vi "Set Winding.vi"(11 "Recipes.Winding":T1) -> (3 "concatenated string":string)   [LabVIEW 2014, in "Programing Logic.lvclass"]
uses:
  Programming Logic/Programing Logic.lvclass
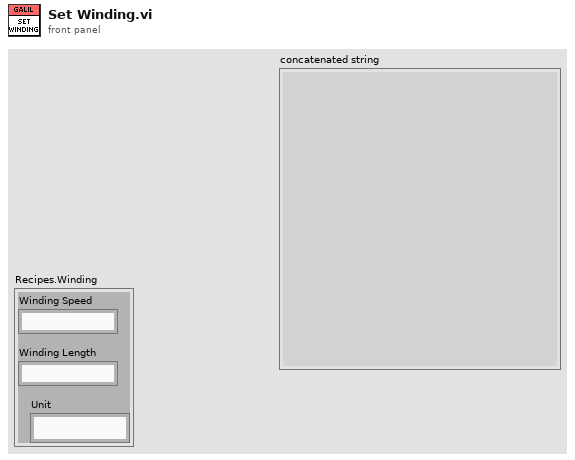
[diagram p1: front panel]
types:
  T1 = cluster{"Winding Speed":string, "Winding Length":string, "Unit":string}
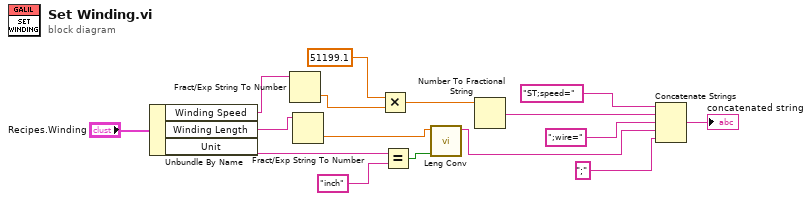
[diagram p0: block diagram]
diagram:
  n1 = Unbundle By Name("Recipes.Winding") -> ("Winding Speed"=w4:string, "Winding Length"=w2:string, "Unit"=w9:string)
  n2 = Fract/Exp String To Number(string=w4) -> (number=w3:dbl)  [unwired: 3 in, 1 out]
  n3 = Fract/Exp String To Number(string=w2) -> (number=w1:dbl)  [unwired: 3 in, 1 out]
  n4 = Multiply(x=51199.1 ("y"), y=w3) -> (x*y=w10:dbl)
  n5 = Equal?(x=w9, y="inch") -> (x = y?=w7:bool)
  n6 = call "Leng Conv.vi"("Unit"=w7, "Winding Length"=w1) -> ("String"=w6:string)  [unwired: 9 in]
  n7 = Number To Fractional String(number=w10) -> (F-format string=w13:string)  [unwired: 3 in]
  n8 = Concatenate Strings("ST;speed=" ("string"), w13, ";wire=" ("string"), w6, ";" ("string")) -> (→"concatenated string":string)
